vi "DO GUI control.vi"(4 "WFGraph Refnum":refnum<vi>, 6 "Sensor Array":refnum<vi>, 7 "Stop Refnum":refnum<vi>, 8 "2nd channel":refnum<vi>, 9 "Dissolved Oxygen":refnum<vi>, 10 "pH":refnum<vi>, 11 "Calibration parameters":refnum<vi>) -> ()   [LabVIEW 2010]
uses:
  global scale array.vi
  DAQ configuration/channel identifier.ctl
  calibration type.ctl
  DAQ configuration/sensor configuration.ctl
  DO.ctl
  pH/pH calibration.ctl
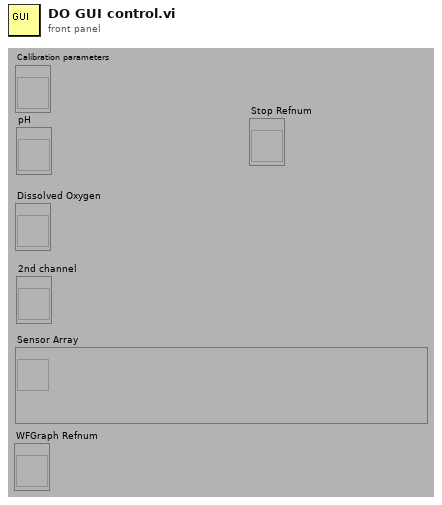
[diagram p1: front panel]
types:
  T1 = cluster{"Port":cluster{"module":u8, "channel":u8}, "calibration type":enum16{"None (raw voltage)", "From File", "Zero voltage", "Edit calibration", "Set calibrated output", "pH", "Dissolved Oxygen", "LVDT calibrator", "NF90 calibrator"}, "name":string}
  T2 = typedef "sensor configuration.ctl" = cluster{"Port":T3, "calibration type":T4, "name":string}
  T3 = typedef "channel identifier.ctl" = u16
  T4 = typedef "calibration type.ctl" = enum16{"None", "Reset to voltage", "Zero voltage", "Set calibrated output", "pH", "Dissolved Oxygen", "LVDT calibrator", "NF90 calibrator"}
  T5 = typedef "calib array.ctl" = T6[]
  T6 = typedef "conversion.ctl" = cluster{"conversion matrix":sgl[][], "units":string, "name":string, "scale type":T7, "offset (volts)":dbl, "second channel":i8, "correspondence table":T8, "offset (physical units)":dbl, "pH scale":T9, "D.O.":T10}
  T7 = typedef "scale type.ctl" = enum16{"Volts", "Polynomial", "Correspondence Table", "pH", "Dissolved Oxygen", "Quadratic"}
  T8 = typedef "correspondence table.ctl" = cluster{"physical units":dbl, "volts":dbl}[]
  T9 = typedef "pH scale.ctl" = cluster{"Buffers":cluster{"Buffer":dbl, "Calibrated":bool, "V/T":dbl}[], "Temperature":dbl}
  T10 = typedef "DO scale.ctl" = cluster{"Temperature":dbl, "K":dbl, "barometric pressure":dbl}
  T11 = cluster{"Buffers":dbl[], "Temperature \ncompensation":bool, "Temperature Index":u32, "Temperature (C)":dbl}
  T12 = cluster{"Controls[][0]":refnum<vi>, "Controls[][1]":refnum<vi>, "Controls[][2]":refnum<vi>, "Controls[][3]":refnum<vi>}
  T13 = cluster{"Temperature Index":u32, "Temperature (C)":dbl, "Temperature\ncompensation":bool, "Barometric Pressure (kPa)":dbl}
  T14 = typedef "DO.ctl" = cluster{"Temperature Index":u32, "Temperature (C)":dbl, "Temperature\ncompensation":bool, "Barometric Pressure (kPa)":dbl}
  T15 = typedef "pH calibration.ctl" = cluster{"Buffers":dbl[], "Temperature \ncompensation":bool, "Temperature Index":u32, "Temperature (C)":dbl}
  T16 = cluster{"Calibrated output":dbl, "2nd channel":T2, "LVDT Index":u32, "Dissolved Oxygen":T14, "pH":T15}
  T17 = cluster{"Controls[][0]":refnum<vi>, "Controls[][1]":refnum<vi>, "Controls[][2]":refnum<vi>, "Controls[][3]":refnum<vi>, "Controls[][4]":refnum<vi>}
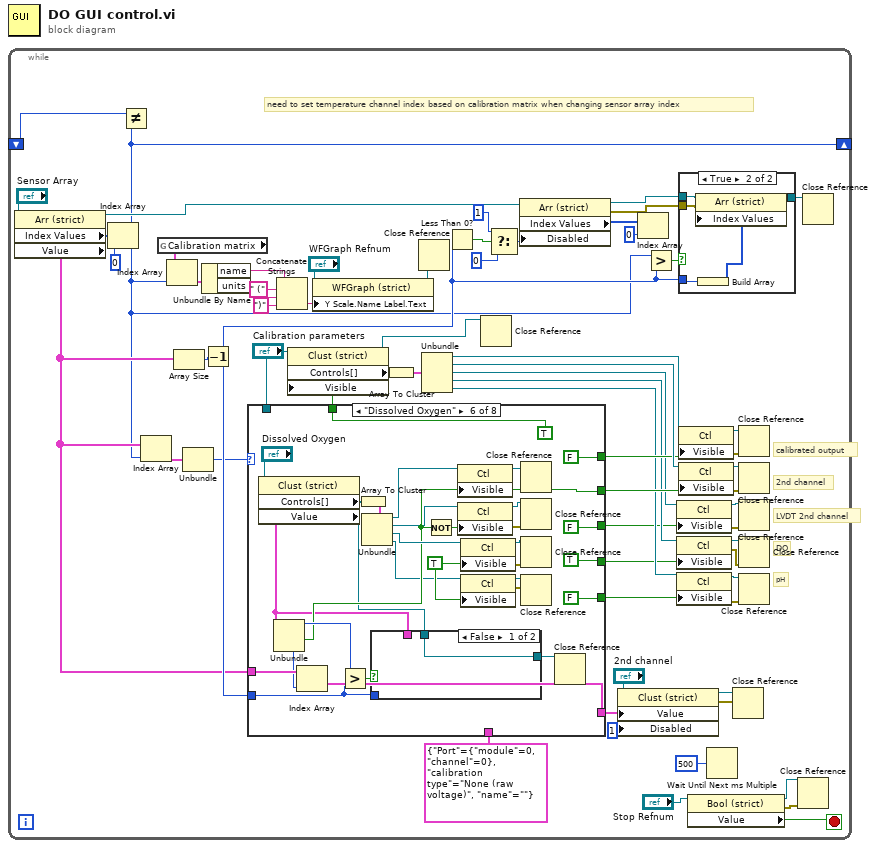
[diagram p0: block diagram]
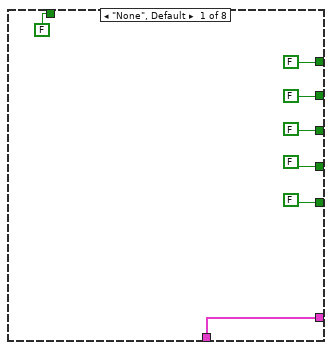
[diagram p3: hidden frame]
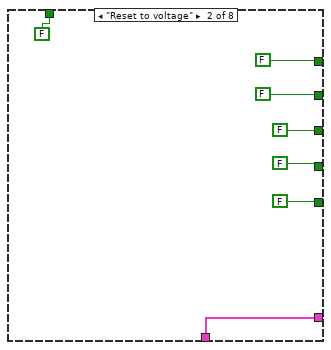
[diagram p4: hidden frame]
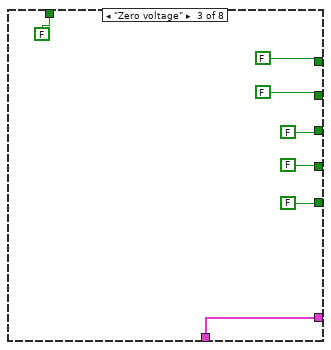
[diagram p5: hidden frame]
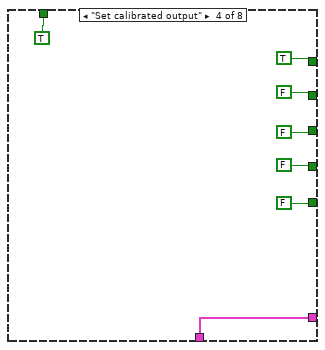
[diagram p6: hidden frame]
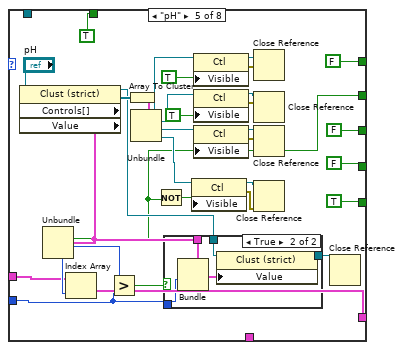
[diagram p7: hidden frame]
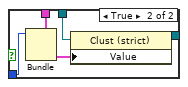
[diagram p9: hidden frame]
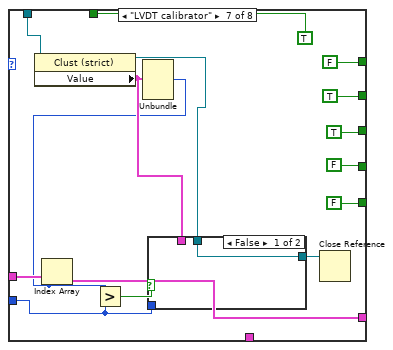
[diagram p10: hidden frame]
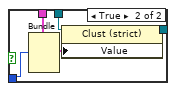
[diagram p11: hidden frame]
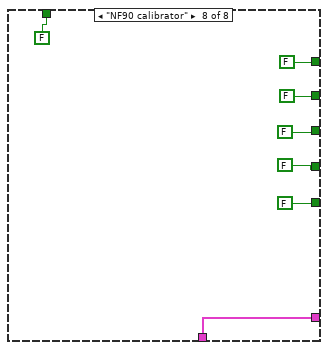
[diagram p12: hidden frame]
diagram:
  n1 = while {
    shift-left: _ -> [w2]
    shift-right: [w1] -> _
    stop <- w26 stop-if-true
    # "need to set temperature channel index based on calibration matrix when changing sensor array index"
    # "DO"
    # "pH"
    # "LVDT 2nd channel"
    # "2nd channel"
    # "calibrated output"
    n2 = property class="Arr (strict)"(reference="Sensor Array") -> (reference out=w19:refnum<vi>, "Index Values"=w29:u32[], "Value"=w31:T2[])  [unwired: 1 in, 1 out]
    n3 = Index Array(array=w29, index=0 ("Index")) -> (element=w1:u32)
    n4 = Not Equal?(x=w2, y=w1) -> ()  [unwired: 1 out]
    n5 = Index Array(array=w31, index=w1) -> (element=w4:T2)
    n6 = global read "global scale array.vi" "Calibration matrix"() -> (w58:T5)
    n7 = Index Array(array=w58, index=w1) -> (element=w57:T6)
    n8 = Array Size(array=w31) -> (size(s)=w48:i32)
    n9 = Unbundle(w4) -> ("calibration type"=w28:T4)  [unwired: 2 out]
    n10 = Unbundle By Name(w57) -> ("name"=w56:string, "units"=w54:string)
    n11 = Decrement(x=w48) -> (x-1=w35:i32)
    n12 = case shown="\"Dissolved Oxygen\"" w28 {
      tunnel: [FALSE ("Visible") FALSE ("Visible") FALSE ("Visible") TRUE ("Visible") FALSE ("Visible") FALSE ("Visible") FALSE ("Visible") FALSE ("Visible")] -> w63
      tunnel: [FALSE ("Visible") FALSE ("Visible") FALSE ("Visible") FALSE ("Visible") w110 w154 TRUE ("Visible") FALSE ("Visible")] -> w62
      tunnel: [FALSE ("Visible") FALSE ("Visible") FALSE ("Visible") TRUE ("Visible") TRUE ("Visible") TRUE ("Visible") TRUE ("Visible") FALSE ("Visible")] -> w60
      tunnel: w31 -> [_ _ _ _ w123 w162 w179 _]
      tunnel: w35 -> [_ _ _ _ w117 w148 w180 _]
      tunnel: [FALSE ("Visible") FALSE ("Visible") FALSE ("Visible") FALSE ("Visible") TRUE ("Visible") FALSE ("Visible") FALSE ("Visible") FALSE ("Visible")] -> w22
      tunnel: [FALSE ("Visible") FALSE ("Visible") FALSE ("Visible") FALSE ("Visible") FALSE ("Visible") TRUE ("Visible") FALSE ("Visible") FALSE ("Visible")] -> w42
      tunnel: [FALSE ("Visible") FALSE ("Visible") FALSE ("Visible") FALSE ("Visible") FALSE ("Visible") FALSE ("Visible") TRUE ("Visible") FALSE ("Visible")] -> w41
      tunnel: [w73 w80 w87 w94 w121 w156 w177 w197] -> w39
      tunnel: "Calibration parameters" -> [_ _ _ _ _ _ w184 _]
      tunnel: T1 {"Port"={"module"=0, "channel"=0}, "calibration type"=enum."None (raw voltage)", "name"=""} ("Cluster") -> [w73 w80 w87 w94 _ _ _ w197]
      frame "None", Default {
      }
      frame "Reset to voltage" {
      }
      frame "Zero voltage" {
      }
      frame "Set calibrated output" {
      }
      frame "pH" {
        n13 = property class="Clust (strict)"(reference="pH") -> (reference out=w125:refnum<vi>, "Controls[]"=w127:refnum<vi>[], "Value"=w122:T11)  [unwired: 1 in, 1 out]
        n14 = Unbundle(w122) -> ("Temperature \ncompensation"=w110:bool, "Temperature Index"=w124:u32)  [unwired: 2 out]
        n15 = Index Array(array=w123, index=w124) -> (element=w121:T2)
        n16 = Greater?(x=w124, y=w117) -> (0:w118:bool)
        n17 = Array To Cluster(array=w127) -> (cluster=w126:T12)
        n18 = Unbundle(w126) -> ("Controls[][0]"=w114:refnum<vi>, "Controls[][1]"=w113:refnum<vi>, "Controls[][2]"=w120:refnum<vi>, "Controls[][3]"=w112:refnum<vi>)
        n19 = Not(x=w110) -> (.not. x?=w111:bool)
        n20 = case shown="True" w118 {
          tunnel: w125 -> [w133 w138]
          tunnel: w122 -> [_ w136]
          tunnel: w117 -> [_ w135]
          tunnel: [w133 w134] -> w109
          frame False {
          }
          frame True {
            n21 = Bundle(cluster=w136, "Temperature Index"=w135) -> (w137:T11)  [unwired: 3 in]
            n22 = property class="Clust (strict)"(reference=w138, "Value"=w137) -> (reference out=w134:refnum<vi>)  [unwired: 1 in, 1 out]
          }
        }
        n23 = property class="Ctl"(reference=w112, "Visible"=w111) -> (reference out=w101:refnum<vi>, error out=w102:errorcluster)  [unwired: 1 in]
        n24 = property class="Ctl"(reference=w114, "Visible"=TRUE) -> (reference out=w108:refnum<vi>, error out=w107:errorcluster)  [unwired: 1 in]
        n25 = property class="Ctl"(reference=w113, "Visible"=TRUE) -> (reference out=w105:refnum<vi>, error out=w106:errorcluster)  [unwired: 1 in]
        n26 = property class="Ctl"(reference=w120, "Visible"=w110) -> (reference out=w103:refnum<vi>, error out=w104:errorcluster)  [unwired: 1 in]
        n27 = Close Reference(reference=w108, error in (no error)=w107) -> ()  [unwired: 1 out]
        n28 = Close Reference(reference=w105, error in (no error)=w106) -> ()  [unwired: 1 out]
        n29 = Close Reference(reference=w103, error in (no error)=w104) -> ()  [unwired: 1 out]
        n30 = Close Reference(reference=w101, error in (no error)=w102) -> ()  [unwired: 1 out]
        n31 = Close Reference(reference=w109) -> ()  [unwired: 1 in, 1 out]
      }
      frame "Dissolved Oxygen" {
        w153 = TRUE ("Visible")
        n32 = property class="Clust (strict)"(reference="Dissolved Oxygen") -> (reference out=w151:refnum<vi>, "Controls[]"=w168:refnum<vi>[], "Value"=w150:T13)  [unwired: 1 in, 1 out]
        n33 = Unbundle(w150) -> ("Temperature Index"=w161:u32, "Temperature\ncompensation"=w154:bool)  [unwired: 2 out]
        n34 = Index Array(array=w162, index=w161) -> (element=w156:T2)
        n35 = Greater?(x=w161, y=w148) -> (0:w149:bool)
        n36 = Array To Cluster(array=w168) -> (cluster=w167:T12)
        n37 = Unbundle(w167) -> ("Controls[][0]"=w166:refnum<vi>, "Controls[][1]"=w165:refnum<vi>, "Controls[][2]"=w155:refnum<vi>, "Controls[][3]"=w152:refnum<vi>)
        n38 = case shown="False" w149 {
          tunnel: w151 -> [w170 w174]
          tunnel: w150 -> [_ w173]
          tunnel: w148 -> [_ w172]
          tunnel: [w170 w171] -> w147
          frame False {
          }
          frame True {
            n39 = Bundle(cluster=w173, "Temperature Index"=w172) -> (w175:T13)  [unwired: 3 in]
            n40 = property class="Clust (strict)"(reference=w174, "Value"=w175) -> (reference out=w171:refnum<vi>)  [unwired: 1 in, 1 out]
          }
        }
        n41 = Not(x=w154) -> (.not. x?=w163:bool)
        n42 = property class="Ctl"(reference=w166, "Visible"=w154) -> (reference out=w145:refnum<vi>, error out=w146:errorcluster)  [unwired: 1 in]
        n43 = property class="Ctl"(reference=w165, "Visible"=w163) -> (reference out=w143:refnum<vi>, error out=w144:errorcluster)  [unwired: 1 in]
        n44 = property class="Ctl"(reference=w155, "Visible"=w153) -> (reference out=w141:refnum<vi>, error out=w142:errorcluster)  [unwired: 1 in]
        n45 = property class="Ctl"(reference=w152, "Visible"=w153) -> (reference out=w139:refnum<vi>, error out=w140:errorcluster)  [unwired: 1 in]
        n46 = Close Reference(reference=w145, error in (no error)=w146) -> ()  [unwired: 1 out]
        n47 = Close Reference(reference=w143, error in (no error)=w144) -> ()  [unwired: 1 out]
        n48 = Close Reference(reference=w141, error in (no error)=w142) -> ()  [unwired: 1 out]
        n49 = Close Reference(reference=w139, error in (no error)=w140) -> ()  [unwired: 1 out]
        n50 = Close Reference(reference=w147) -> ()  [unwired: 1 in, 1 out]
      }
      frame "LVDT calibrator" {
        n51 = property class="Clust (strict)"(reference=w184) -> (reference out=w183:refnum<vi>, "Value"=w182:T16)  [unwired: 1 in, 1 out]
        n52 = Unbundle(w182) -> ("LVDT Index"=w178:u32)  [unwired: 4 out]
        n53 = Index Array(array=w179, index=w178) -> (element=w177:T2)
        n54 = Greater?(x=w178, y=w180) -> (0:w181:bool)
        n55 = case shown="False" w181 {
          tunnel: w183 -> [w191 w196]
          tunnel: w182 -> [_ w194]
          tunnel: w180 -> [_ w193]
          tunnel: [w191 w192] -> w176
          frame False {
          }
          frame True {
            n56 = Bundle(cluster=w194, "LVDT Index"=w193) -> (w195:T16)  [unwired: 4 in]
            n57 = property class="Clust (strict)"(reference=w196, "Value"=w195) -> (reference out=w192:refnum<vi>)  [unwired: 1 in, 1 out]
          }
        }
        n58 = Close Reference(reference=w176) -> ()  [unwired: 1 in, 1 out]
      }
      frame "NF90 calibrator" {
      }
    }
    n59 = Concatenate Strings(w56, " (" ("Substring"), w54, ")" ("Substring")) -> (w52:string)
    n60 = property class="Clust (strict)"(reference="Calibration parameters", "Visible"=w60) -> (reference out=w15:refnum<vi>, "Controls[]"=w61:refnum<vi>[])  [unwired: 1 in, 1 out]
    n61 = property class="WFGraph (strict)"(reference="WFGraph Refnum", "Y Scale.Name Label.Text"=w52) -> (reference out=w21:refnum<vi>)  [unwired: 1 in, 1 out]
    n62 = Array To Cluster(array=w61) -> (cluster=w64:T17)
    n63 = Close Reference(reference=w21) -> ()  [unwired: 1 in, 1 out]
    n64 = Unbundle(w64) -> ("Controls[][0]"=w66:refnum<vi>, "Controls[][1]"=w65:refnum<vi>, "Controls[][2]"=w45:refnum<vi>, "Controls[][3]"=w44:refnum<vi>, "Controls[][4]"=w43:refnum<vi>)
    n65 = Less Than 0?(x=w35) -> (x < 0?=w36:bool)
    n66 = Close Reference(reference=w15) -> ()  [unwired: 1 in, 1 out]
    n67 = Select(t=u8 1 ("Disabled"), s=w36, f=u8 0 ("Disabled")) -> (s? t:f=w32:u8)
    n68 = property class="Arr (strict)"(reference=w19, "Disabled"=w32) -> (reference out=w51:refnum<vi>, error out=w50:errorcluster, "Index Values"=w37:u32[])  [unwired: 1 in]
    n69 = property class="Clust (strict)"(reference="2nd channel", "Value"=w39, "Disabled"=u8 1) -> (reference out=w17:refnum<vi>, error out=w16:errorcluster)  [unwired: 1 in]
    n70 = Index Array(array=w37, index=0 ("Index")) -> ()  [unwired: 1 out]
    n71 = Greater?(x=w1, y=w35) -> (0:w38:bool)
    n72 = property class="Ctl"(reference=w45, "Visible"=w41) -> (reference out=w9:refnum<vi>, error out=w10:errorcluster)  [unwired: 1 in]
    n73 = property class="Ctl"(reference=w44, "Visible"=w42) -> (reference out=w7:refnum<vi>, error out=w8:errorcluster)  [unwired: 1 in]
    n74 = property class="Ctl"(reference=w43, "Visible"=w22) -> (reference out=w5:refnum<vi>, error out=w6:errorcluster)  [unwired: 1 in]
    n75 = case shown="True" w38 {
      tunnel: w51 -> [w67 w72]
      tunnel: w50 -> [_ w71]
      tunnel: w35 -> [_ w70]
      tunnel: [w67 w68] -> w18
      frame False {
      }
      frame True {
        n76 = Build Array(w70) -> (w69:i32[])
        n77 = property class="Arr (strict)"(reference=w72, error in=w71, "Index Values"=w69) -> (reference out=w68:refnum<vi>)  [unwired: 1 out]
      }
    }
    n78 = property class="Ctl"(reference=w66, "Visible"=w63) -> (reference out=w13:refnum<vi>, error out=w14:errorcluster)  [unwired: 1 in]
    n79 = property class="Ctl"(reference=w65, "Visible"=w62) -> (reference out=w11:refnum<vi>, error out=w12:errorcluster)  [unwired: 1 in]
    n80 = property class="Bool (strict)"(reference="Stop Refnum") -> (reference out=w24:refnum<vi>, error out=w25:errorcluster, "Value"=w26:bool)  [unwired: 1 in]
    n81 = Wait Until Next ms Multiple(millisecond multiple=u32 500) -> ()  [unwired: 1 out]
    n82 = Close Reference(reference=w17, error in (no error)=w16) -> ()  [unwired: 1 out]
    n83 = Close Reference(reference=w13, error in (no error)=w14) -> ()  [unwired: 1 out]
    n84 = Close Reference(reference=w11, error in (no error)=w12) -> ()  [unwired: 1 out]
    n85 = Close Reference(reference=w9, error in (no error)=w10) -> ()  [unwired: 1 out]
    n86 = Close Reference(reference=w7, error in (no error)=w8) -> ()  [unwired: 1 out]
    n87 = Close Reference(reference=w5, error in (no error)=w6) -> ()  [unwired: 1 out]
    n88 = Close Reference(reference=w24, error in (no error)=w25) -> ()  [unwired: 1 out]
    n89 = Close Reference(reference=w18) -> ()  [unwired: 1 in, 1 out]
  }
